vi "10.5.vi"() -> ()   [LabVIEW 2019]
panel:
  out "loop time":u32
  out "for loop array":dbl[](array[numeric])
  in  "number of elements":dbl
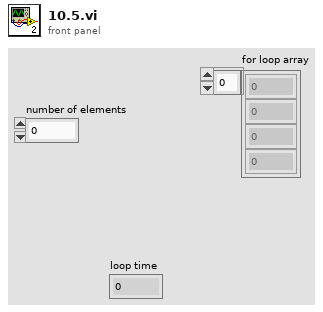
[diagram p1: front panel]
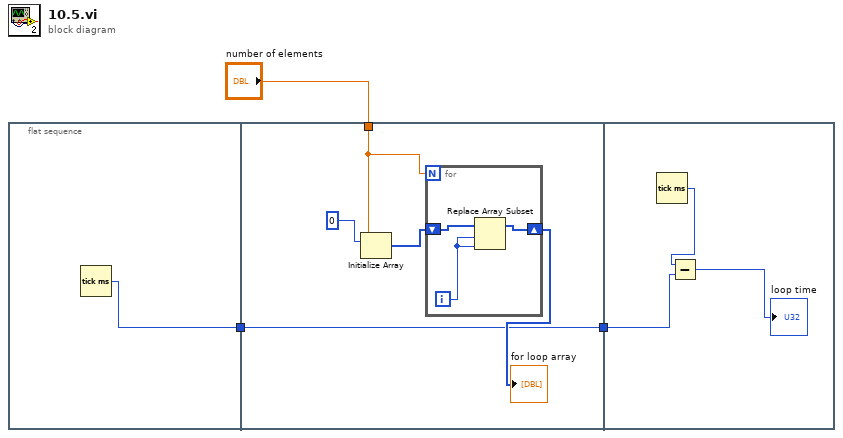
[diagram p0: block diagram]
diagram:
  n1 = flat-sequence {
    tunnel: [w4] -> w1
    tunnel: "number of elements" -> [w7]
    tunnel: [w5] -> w2
    tunnel: w1 -> [w5]
    tunnel: w2 -> [w15]
    frame #0 {
      n2 = Tick Count (ms)() -> (millisecond timer value=w4:u32)
    }
    frame #1 {
      n3 = Initialize Array(0, w7) -> (w8:i32[])
      n4 = for {
        N: w7 -> [_]
        shift-right: [w10] -> w6
        shift-left: w8 -> [w11]
        i -> [w12]
        n5 = Replace Array Subset(array=w11, new element=w12, index=w12) -> (w10:i32[])
      }
      "for loop array" <- w6
    }
    frame #2 {
      n6 = Tick Count (ms)() -> (millisecond timer value=w14:u32)
      n7 = Subtract(x=w14, y=w15) -> (x-y=→"loop time":u32)
    }
  }
